vi "UnInit.vi"(2 "Container State":T1 caption="容器状态", 3 "Display State":T2 caption="显示状态") -> ()   [LabVIEW 2011, in "WaveFormGraph.xctl"]
uses:
  WaveFormGraph.xctl
  State.ctl
  F:/Program Files/National Instruments/LabVIEW 2011/resource/importtools/Common/Event/NISAST Event.lvclass
  CursorPosQueueCluster.ctl
  <vilib>/_xctls/Container State.ctl
  <vilib>/_xctls/XControlSupport.lvlib
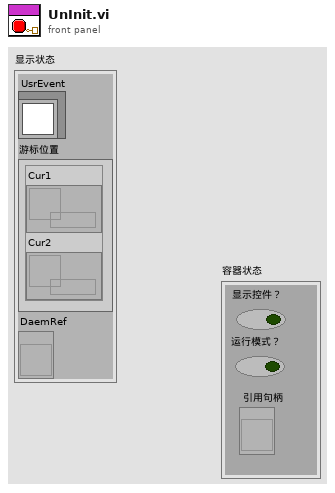
[diagram p1: front panel]
types:
  T1 = typedef "XControlSupport.lvlib/Container State.ctl" = cluster{"Indicator?":bool, "Run Mode?":bool, " Refnum":refnum<vi>}
  T2 = typedef "WaveFormGraph.xctl/State.ctl" = cluster{"UsrEvent":refnum<class "NISAST Event.lvclass">, "游标位置":T3, "DaemRef":refnum<vi>}
  T3 = typedef "CursorPosQueueCluster.ctl" = cluster{"Cur1":refnum<queue>, "Cur2":refnum<queue>}
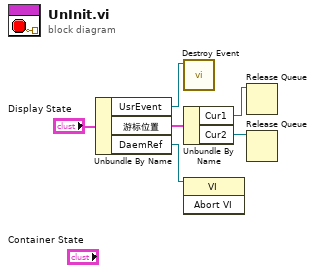
[diagram p0: block diagram]
diagram:
  n1 = Unbundle By Name("Display State") -> ("UsrEvent"=w5:refnum<class "NISAST Event.lvclass">, "游标位置"=w4:T3, "DaemRef"=w1:refnum<vi>)
  n2 = call-dynamic "Destroy Event.vi"("Event in"=w5) -> ()  [unwired: 9 in, 2 out]
  n3 = Unbundle By Name(w4) -> ("Cur1"=w3:refnum<queue>, "Cur2"=w2:refnum<queue>)
  n4 = invoke class="VI" method="Abort VI"(reference=w1) -> ()  [unwired: 2 in, 3 out]
  n5 = Release Queue(queue=w3) -> ()  [unwired: 2 in, 3 out]
  n6 = Release Queue(queue=w2) -> ()  [unwired: 2 in, 3 out]
